vi "SDT_ReadSetUpBlock.vi"(8 "error in":errorcluster, 10 "bhfile_header":T1 {"chksum" format="x%x"; "header_valid" format="x%x"}, 11 "SDTFileRefnum":refnum<file>) -> (0 "error out":errorcluster, 1 "SetUp":string, 2 "FileInfo":string, 3 "SDTFileRefnum":refnum<file>, 4 "SetUpLength":i32, 5 "MagicNum":u16 format="%x", 6 "BinarySetup_length":u16)   [LabVIEW 2019]
doc: "This VI is a SubVI to SDT_ReadFile.vi . It reads the ASCII- and first part of the binary-SetUp block in a SDT-file from disc.\nSee also a different approach at \\Public\\Data\\SPC Files\\SPCGetTimeScaleFromSETfile.vi.\nFor a description of the *.sdt file format see: SPC_data_file_structure.h\n\ninfo@becker-hickl.com"
uses:
  SPC_Controls/WFParam.ctl
  SPC_Controls/SPCBinHdrExt.ctl
  SPC_Controls/SPCBinHdr.ctl
  SPC_Controls/BHBinHdr.ctl
  SPC_Controls/bhfile_header.ctl
panel:
  out "BHBinHdr":T2
  out "SPCBinHdr":T3
  out "SPCBinHdrExt":T4
  out "WFParam":T5
  out "chksumTopUp":u16 format="%x"
  out "BinarySetUp":string
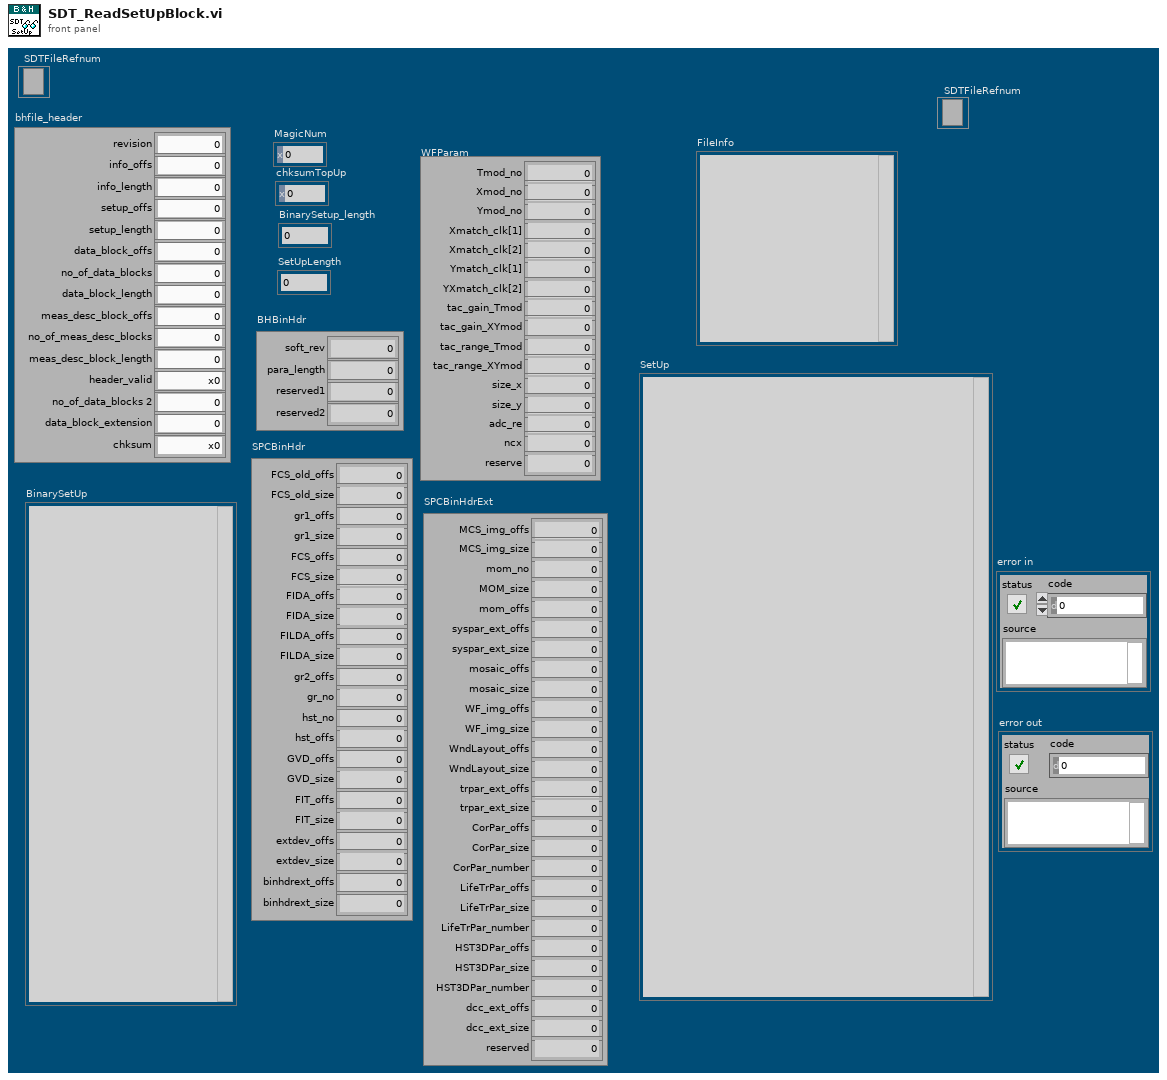
[diagram p1: front panel]
types:
  T1 = typedef "bhfile_header.ctl" = cluster{"revision":i16, "info_offs":i32, "info_length":i16, "setup_offs":i32, "setup_length":u16, "data_block_offs":i32, "no_of_data_blocks":i16, "data_block_length":u32, "meas_desc_block_offs":i32, "no_of_meas_desc_blocks":i16, "meas_desc_block_length":i16, "header_valid":u16, "no_of_data_blocks 2":u32, "data_block_extension":u16, "chksum":u16}
  T2 = typedef "BHBinHdr.ctl" = cluster{"soft_rev":u32, "para_length":u32, "reserved1":u32, "reserved2":u16}
  T3 = typedef "SPCBinHdr.ctl" = cluster{"FCS_old_offs":u32, "FCS_old_size":u32, "gr1_offs":u32, "gr1_size":u32, "FCS_offs":u32, "FCS_size":u32, "FIDA_offs":u32, "FIDA_size":u32, "FILDA_offs":u32, "FILDA_size":u32, "gr2_offs":u32, "gr_no":u16, "hst_no":u16, "hst_offs":u32, "GVD_offs":u32, "GVD_size":u16, "FIT_offs":u16, "FIT_size":u16, "extdev_offs":u16, "extdev_size":u16, "binhdrext_offs":u32, "binhdrext_size":u16}
  T4 = typedef "SPCBinHdrExt.ctl" = cluster{"MCS_img_offs":u32, "MCS_img_size":u32, "mom_no":u16, "MOM_size":u16, "mom_offs":u32, "syspar_ext_offs":u32, "syspar_ext_size":u32, "mosaic_offs":u32, "mosaic_size":u32, "WF_img_offs":u32, "WF_img_size":u16, "WndLayout_offs":u32, "WndLayout_size":u16, "trpar_ext_offs":u32, "trpar_ext_size":u16, "CorPar_offs":u32, "CorPar_size":u16, "CorPar_number":u16, "LifeTrPar_offs":u32, "LifeTrPar_size":u16, "LifeTrPar_number":u16, "HST3DPar_offs":u32, "HST3DPar_size":u16, "HST3DPar_number":u16, "dcc_ext_offs":u32, "dcc_ext_size":u16, "reserved":u16}
  T5 = typedef "WFParam.ctl" = cluster{"Tmod_no":i16, "Xmod_no":i16, "Ymod_no":i16, "Xmatch_clk[1]":i16, "Xmatch_clk[2]":i16, "Ymatch_clk[1]":i16, "YXmatch_clk[2]":i16, "tac_gain_Tmod":i16, "tac_gain_XYmod":i16, "tac_range_Tmod":sgl, "tac_range_XYmod":sgl, "size_x":i16, "size_y":i16, "adc_re":i16, "ncx":i16, "reserve":i16}
  T6 = enum16{"big-endian, network order", "native, host order", "little-endian"}
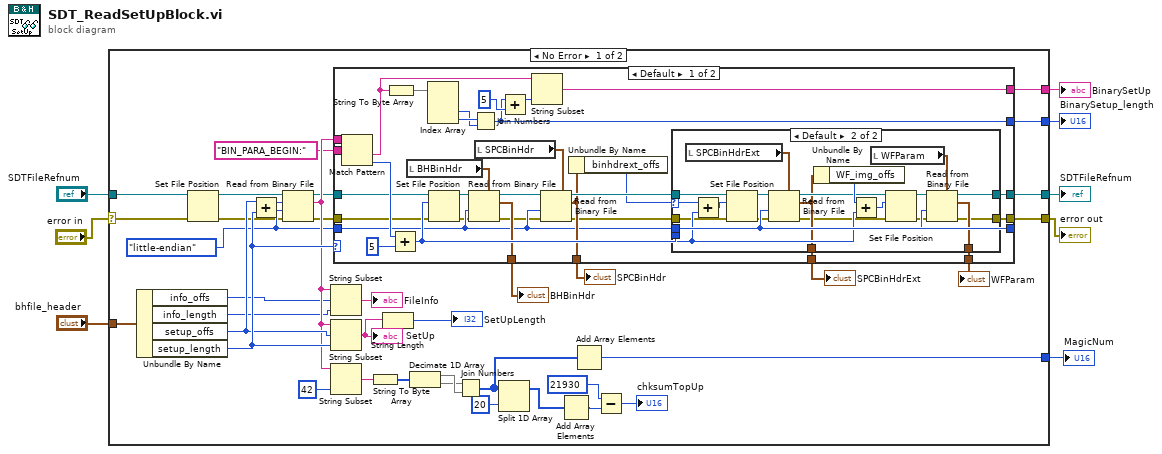
[diagram p0: block diagram]
diagram:
  n1 = case shown="No Error" "error in" {
    selector: "error in" -> [w13 w104]
    tunnel: [w42 _] -> w8
    tunnel: [w41 _] -> w7
    tunnel: "bhfile_header" -> [w21 _]
    tunnel: "SDTFileRefnum" -> [w20 w103]
    tunnel: [w19 w103] -> w4
    tunnel: [w10 w104] -> w2
    tunnel: [w9 _] -> w1
    frame No Error {
      w14 = T6."little-endian" ("byte order (0:big-endian, network order)")
      n2 = Unbundle By Name(w21) -> ("info_offs"=w24:i32, "info_length"=w25:i16, "setup_offs"=w43:i32, "setup_length"=w44:u16)
      n3 = Set File Position(refnum=w20, error in=w13) -> (refnum out=w26:refnum<file>, error out=w12:errorcluster)  [unwired: 2 in]
      n4 = Add(x=w43, y=w44) -> (x+y=w27:i32)
      n5 = Read from Binary File(8:w12, 9:w14, 10:w27, 11:w26) -> (0:w11:errorcluster, 2:w29:string, 3:w28:refnum<file>)  [unwired: 2 in, 1 out]
      n6 = String Subset(string=w29, offset (0)=w24, length (rest)=w25) -> (substring=→"FileInfo":string)
      n7 = String Subset(string=w29, offset (0)=w43, length (rest)=w44) -> (substring=w45:string)
      "SetUp" <- w45
      n8 = String Subset(string=w29, length (rest)=42 ("length (rest)")) -> (substring=w31:string)  [unwired: 1 in]
      n9 = case shown="Default" w44 {
        tunnel: "BIN_PARA_BEGIN:" ("regular expression") -> [w77 _]
        tunnel: [w63 w102] -> w19
        tunnel: w28 -> [w62 w102]
        tunnel: w14 -> [w56 w101]
        tunnel: w29 -> [w61 _]
        tunnel: [w60 _] -> w15
        tunnel: [w59 _] -> w16
        tunnel: [w58 _] -> w17
        tunnel: [w57 _] -> w18
        tunnel: [w56 w101] -> _
        tunnel: [w55 _] -> w41
        tunnel: [w54 _] -> w42
        tunnel: w11 -> [w51 w100]
        tunnel: [w47 w100] -> w10
        frame Default {
          n10 = Match Pattern(string=w61, regular expression=w77) -> (after substring=w73:string, offset past match=w69:i32)  [unwired: 1 in, 2 out]
          n11 = String To Byte Array(string=w73) -> (unsigned byte array=w76:u8[])
          n12 = Add(x=w69, y=5) -> (x+y=w64:i32)
          n13 = local read "BHBinHdr"() -> (w53:T2)
          n14 = Index Array(array=w76) -> (element #2=w74:u8, element #3=w75:u8)  [unwired: 3 in, 1 out]
          n15 = Set File Position(offset (in bytes) (0)=w64, refnum=w62, error in=w51) -> (refnum out=w70:refnum<file>, error out=w50:errorcluster)  [unwired: 1 in]
          n16 = Read from Binary File(5:w53, 8:w50, 9:w56, 11:w70) -> (0:w49:errorcluster, 2:w57:T2, 3:w67:refnum<file>)  [unwired: 2 in, 1 out]
          n17 = Join Numbers(hi=w75, lo=w74) -> ((hi.lo)=w55:u16)
          n18 = local read "SPCBinHdr"() -> (w52:T3)
          n19 = Add(x=w55, y=u16 5) -> (x+y=w72:u16)
          n20 = String Subset(string=w73, length (rest)=w72) -> (substring=w54:string)  [unwired: 1 in]
          n21 = Read from Binary File(5:w52, 8:w49, 9:w56, 11:w67) -> (0:w48:errorcluster, 2:w58:T3, 3:w66:refnum<file>)  [unwired: 2 in, 1 out]
          n22 = Unbundle By Name(w58) -> ("binhdrext_offs"=w65:u32)
          n23 = case shown="Default" w65 {
            selector: w65 -> [_ w94]
            tunnel: w66 -> [w78 w98]
            tunnel: w64 -> [_ w91]
            tunnel: [w78 w90] -> w63
            tunnel: [_ w89] -> w60
            tunnel: [_ w88] -> w59
            tunnel: w56 -> [_ w87]
            tunnel: w48 -> [w79 w84]
            tunnel: [w79 w80] -> w47
            frame 0 {
            }
            frame Default {
              n24 = local read "SPCBinHdrExt"() -> (w86:T4)
              n25 = Add(x=w94, y=w91) -> (x+y=w93:u32)
              n26 = Set File Position(offset (in bytes) (0)=w93, refnum=w98, error in=w84) -> (refnum out=w99:refnum<file>, error out=w83:errorcluster)  [unwired: 1 in]
              n27 = Read from Binary File(5:w86, 8:w83, 9:w87, 11:w99) -> (0:w82:errorcluster, 2:w88:T4, 3:w95:refnum<file>)  [unwired: 2 in, 1 out]
              n28 = Unbundle By Name(w88) -> ("WF_img_offs"=w96:u32)
              n29 = Add(x=w96, y=w91) -> (x+y=w92:u32)
              n30 = local read "WFParam"() -> (w85:T5)
              n31 = Set File Position(offset (in bytes) (0)=w92, refnum=w95, error in=w82) -> (refnum out=w97:refnum<file>, error out=w81:errorcluster)  [unwired: 1 in]
              n32 = Read from Binary File(5:w85, 8:w81, 9:w87, 11:w97) -> (0:w80:errorcluster, 2:w89:T5, 3:w90:refnum<file>)  [unwired: 2 in, 1 out]
            }
          }
        }
        frame 0 {
        }
      }
      "BHBinHdr" <- w18
      "SPCBinHdr" <- w17
      "SPCBinHdrExt" <- w16
      "WFParam" <- w15
      n33 = String To Byte Array(string=w31) -> (unsigned byte array=w32:u8[])
      n34 = String Length(string=w45) -> (length=→"SetUpLength":i32)
      n35 = Decimate 1D Array(w32) -> (w34:u8[], w33:u8[])
      n36 = Join Numbers(hi=w33, lo=w34) -> ((hi.lo)=w36:u16[])
      n37 = Split 1D Array(array=w36, index=20) -> (first subarray=w37:u16[])  [unwired: 1 out]
      n38 = Add Array Elements(numeric array=w37) -> (sum=w38:u16)
      n39 = Add Array Elements(numeric array=w36) -> (sum=w9:u16)
      n40 = Subtract(x=u16 21930 ("y"), y=w38) -> (x-y=→"chksumTopUp":u16)
    }
    frame Error {
    }
  }
  "BinarySetup_length" <- w7
  "BinarySetUp" <- w8
  "SDTFileRefnum" <- w4
  "error out" <- w2
  "MagicNum" <- w1
